vi "GraphFormatting.vi"(4 "Error In":errorcluster, 5 "GraphIndex":T1, 6 "VoltageChannels1(0to15)":dbl[](array[numeric])=[1.0, 1.0], 7 "WBridgeChannels":dbl[](array[numeric])=[1000.0, 1000.0]) -> (0 "Error Out":errorcluster, 2 "Graph2Data":dbl[][](array[numeric]), 3 "Graph1Data":dbl[][](array[numeric]))   [LabVIEW 2015]
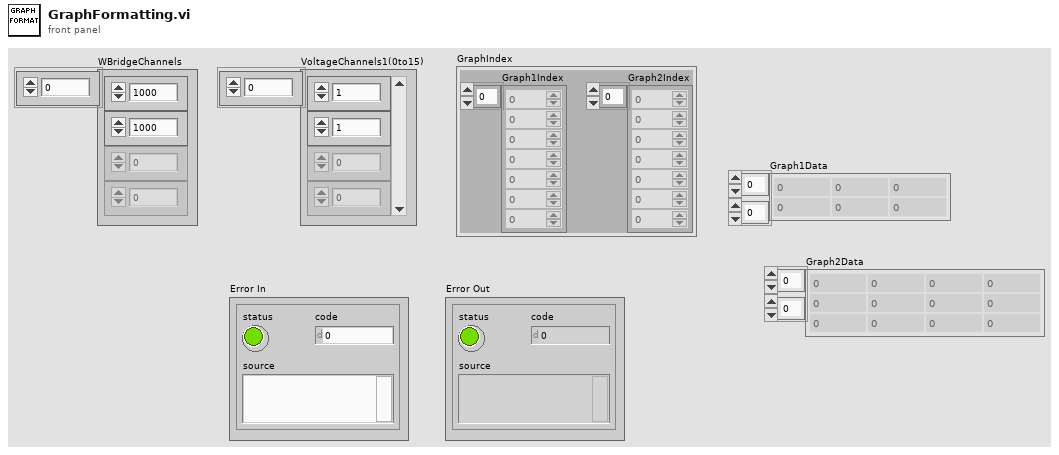
[diagram p1: front panel]
types:
  T1 = cluster{"Graph2Index":i32[], "Graph1Index":i32[]}
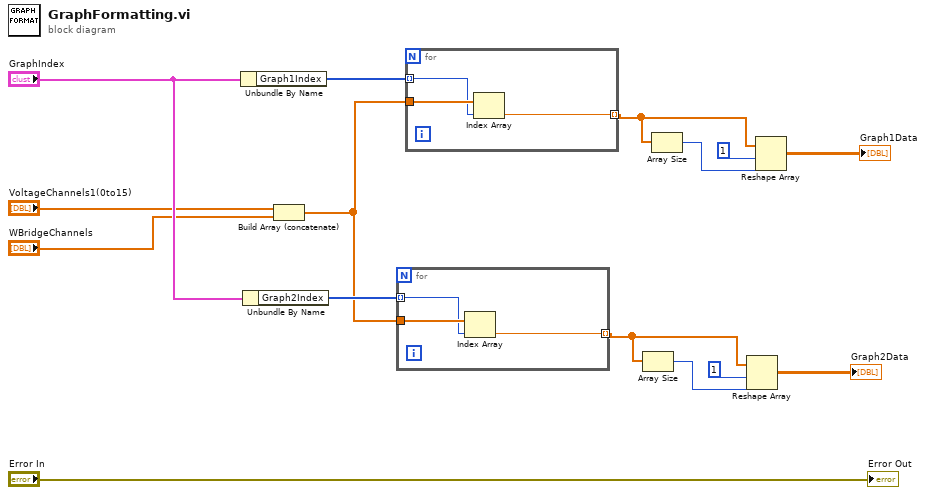
[diagram p0: block diagram]
diagram:
  n1 = Unbundle By Name("GraphIndex") -> ("Graph1Index"=w15:i32[])
  n2 = Unbundle By Name("GraphIndex") -> ("Graph2Index"=w7:i32[])
  n3 = Build Array (concatenate)("VoltageChannels1(0to15)", "WBridgeChannels") -> (w6:dbl[])
  n4 = for {
    tunnel: w7 -> [w17] mode=indexing
    tunnel: w6 -> [w18]
    tunnel: [w16] -> w10 mode=indexing
    n5 = Index Array(array=w18, index=w17) -> (element=w16:dbl)
  }
  n6 = for {
    tunnel: w15 -> [w20] mode=indexing
    tunnel: w6 -> [w21]
    tunnel: [w19] -> w12 mode=indexing
    n7 = Index Array(array=w21, index=w20) -> (element=w19:dbl)
  }
  n8 = Array Size(array=w10) -> (size(s)=w9:i32)
  n9 = Array Size(array=w12) -> (size(s)=w13:i32)
  n10 = Reshape Array(w10, 1 ("taille de la dimension"), w9) -> (→"Graph2Data":dbl[][])
  n11 = Reshape Array(w12, 1 ("taille de la dimension"), w13) -> (→"Graph1Data":dbl[][])
  "Error Out" <- "Error In"
